vi "数的位数.vi"(1 "Mode":enum16{"DEC", "HEX", "OCT", "BIN"}(ring), 3 "Number In":i32) -> (0 "Digits":u8)   [LabVIEW 2015]
doc: "Changes a double's value to '0' if it is 'NaN'.\n\nFreeware from Moore Good Ideas, www.mooregoodideas.com. Do not remove this line."
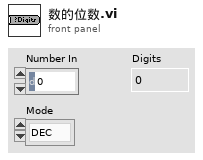
[diagram p1: front panel]
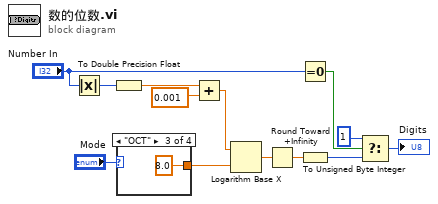
[diagram p0: block diagram]
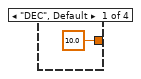
[diagram p2: hidden frame]
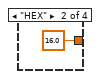
[diagram p3: hidden frame]
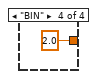
[diagram p4: hidden frame]
diagram:
  n1 = Absolute Value(x="Number In") -> (abs(x)=w12:i32)
  n2 = To Double Precision Float(number=w12) -> (double precision float=w1:dbl)
  n3 = case shown="\"OCT\"" "Mode" {
    tunnel: [10.0 ("y") 16.0 ("y") 8.0 ("y") 2.0 ("y")] -> w10
    frame "DEC", Default {
    }
    frame "HEX" {
    }
    frame "OCT" {
    }
    frame "BIN" {
    }
  }
  n4 = Add(x=w1, y=0.001) -> (x+y=w9:dbl)
  n5 = Logarithm Base X(1:w10, 2:w9) -> (0:w8:dbl)
  n6 = Round Toward +Infinity(x=w8) -> (ceil(x): smallest int >= x=w7:dbl)
  n7 = Equal To 0?(x="Number In") -> (x = 0?=w5:bool)
  n8 = To Unsigned Byte Integer(number=w7) -> (unsigned 8bit integer=w3:u8)
  n9 = Select(t=u8 1 ("Digits"), s=w5, f=w3) -> (s? t:f=→"Digits":u8)
